vi "Extended.BuildSysexMsgI2CReadWrite.vi"(4 "use10BitsAddressMode?":bool, 6 "useAutoRestartTransmission?":bool, 7 "Read/Write Mode":T1(ring), 8 "error in":errorcluster, 9 "Register":u16 format="%.0x", 10 "I2C Write Data":u8[](array[numeric]) format="%x", 11 "Slave Address":u8 format="%x") -> (0 "error out":errorcluster, 1 "ReplyLength":i32=-1, 2 "ReplyFirstByte":T2=224 items=["ANALOG_IO_MESSAGE"=224, "DIGITAL_IO_MESSAGE"=144, "REPORT_ANALOG_PIN"=192, "REPORT_DIGITAL_PORT"=208, "START_SYSEX"=240, "END_SYSEX"=247, "SET_PIN_MODE"=244, "SET_DIGITAL_PIN_VALUE"=245, "PROTOCOL_VERSION"=249, "SYSTEM_RESET"=255, "SYSEX.EXTENDED_ID"=0, "SYSEX.RESERVED_USER_COMMANDs"=1, "SYSEX.ANALOG_MAPPING_QUERY"=105, "SYSEX.ANALOG_MAPPING_RESPONSE"=106, "SYSEX.CAPABILITY_QUERY"=107, "SYSEX.CAPABILITY_RESPONSE"=108, "SYSEX.PIN_STATE_QUERY"=109, "SYSEX.PIN_STATE_RESPONSE"=110, "SYSEX.REPORT_FIRMWARE"=121, "SYSEX.EXTENDED_ANALOG"=111, "SYSEX.STRING_DATA"=113, "SYSEX.REALTIME"=127, "SYSEX.NON_REALTIME"=126, "SYSEX.SAMPLING_INTERVAL"=122], 3 "I2CRequestMessage":u8[](array[numeric]) format="%x")   [LabVIEW 2020, in "FirmataClient.lvlib"]
doc: "Builds a message according to the Firmata Protocol Requirements. \n- https://github.com/firmata/protocol\n- https://github.com/firmata/protocol/blob/master/protocol.md"
uses:
  FirmataClient.lvlib
  controls/FirmataProtocolConstants.ctl
  8aab0f93-2f9c-4515-bdca-9512dbea522e.vi
  147f2e90-8315-44ff-bc99-ac74707c4f68.vi
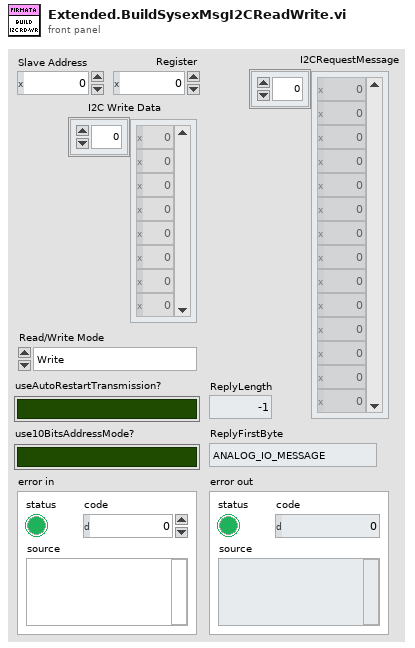
[diagram p1: front panel]
types:
  T1 = enum16{"Write", "Read Once", "Read Continuously", "Stop Continuous Reading"}
  T2 = typedef "FirmataClient.lvlib/FirmataProtocolConstants.ctl" = u16
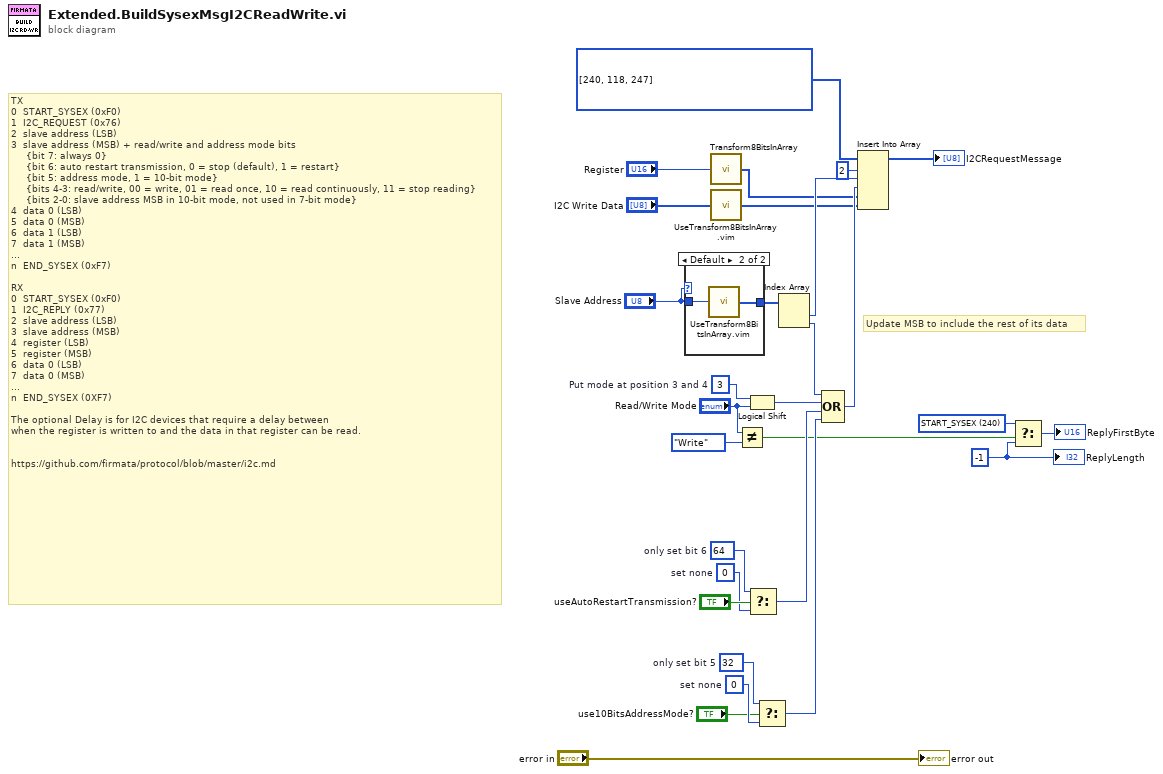
[diagram p0: block diagram]
diagram:
  w9 = T2 240 items=["ANALOG_IO_MESSAGE"=224, "DIGITAL_IO_MESSAGE"=144, "REPORT_ANALOG_PIN"=192, "REPORT_DIGITAL_PORT"=208, "START_SYSEX"=240, "END_SYSEX"=247, "SET_PIN_MODE"=244, "SET_DIGITAL_PIN_VALUE"=245, "PROTOCOL_VERSION"=249, "SYSTEM_RESET"=255, "SYSEX.EXTENDED_ID"=0, "SYSEX.RESERVED_USER_COMMANDs"=1, "SYSEX.ANALOG_MAPPING_QUERY"=105, "SYSEX.ANALOG_MAPPING_RESPONSE"=106, "SYSEX.CAPABILITY_QUERY"=107, "SYSEX.CAPABILITY_RESPONSE"=108, "SYSEX.PIN_STATE_QUERY"=109, "SYSEX.PIN_STATE_RESPONSE"=110, "SYSEX.REPORT_FIRMWARE"=121, "SYSEX.EXTENDED_ANALOG"=111, "SYSEX.STRING_DATA"=113, "SYSEX.REALTIME"=127, "SYSEX.NON_REALTIME"=126, "SYSEX.SAMPLING_INTERVAL"=122, "FEATURES.SYSEX.I2C_READ_WRITE"=118, "FEATURES.SYSEX.I2C_REPLY"=119, "FEATURES.SYSEX.I2C_CONFIG"=120] ("ReplyFirstByte")
  w16 = u8 0  # set none
  w15 = u8 32  # only set bit 5
  w18 = u8 0  # set none
  w19 = u8 64  # only set bit 6
  w11 = u8 3  # Put mode at position 3 and 4
  w8 = -1 ("ReplyLength")
  w27 = T2[] [240, 118, 247] items=["ANALOG_IO_MESSAGE"=224, "DIGITAL_IO_MESSAGE"=144, "REPORT_ANALOG_PIN"=192, "REPORT_DIGITAL_PORT"=208, "START_SYSEX"=240, "END_SYSEX"=247, "SET_PIN_MODE"=244, "SET_DIGITAL_PIN_VALUE"=245, "PROTOCOL_VERSION"=249, "SYSTEM_RESET"=255, "SYSEX.EXTENDED_ID"=0, "SYSEX.RESERVED_USER_COMMANDs"=1, "SYSEX.ANALOG_MAPPING_QUERY"=105, "SYSEX.ANALOG_MAPPING_RESPONSE"=106, "SYSEX.CAPABILITY_QUERY"=107, "SYSEX.CAPABILITY_RESPONSE"=108, "SYSEX.PIN_STATE_QUERY"=109, "SYSEX.PIN_STATE_RESPONSE"=110, "SYSEX.REPORT_FIRMWARE"=121, "SYSEX.EXTENDED_ANALOG"=111, "SYSEX.STRING_DATA"=113, "SYSEX.REALTIME"=127, "SYSEX.NON_REALTIME"=126, "SYSEX.SAMPLING_INTERVAL"=122, "FEATURES.SYSEX.I2C_READ_WRITE"=118, "FEATURES.SYSEX.I2C_REPLY"=119, "FEATURES.SYSEX.I2C_CONFIG"=120]
  # "Update MSB to include the rest of its data"
  # "TX\n0  START_SYSEX (0xF0)\n1  I2C_REQUEST (0x76)\n2  slave address (LSB)\n3  slave address (MSB) + read/write and address mode bits\n     {bit 7: always 0}\n     {bit 6: auto restart transmission, 0 = stop (default), 1 = restart}\n     {bit 5: address mode, 1 = 10-bit mode}\n     {bits 4-3: read/write, 00 = write, 01 = read once, 10 = read continuously, 11 = stop reading}\n     {bits 2-0: slave address MSB in 10-bit mode, not used in 7-bit mode}\n4  data 0 (LSB)\n5  data 0 (MSB)\n6  data 1 (LSB)\n7  data 1 (MSB)\n...\nn  END_SYSEX (0xF7)\n\nRX\n0  START_SYSEX (0xF0)\n1  I2C_REPLY (0x77)\n2  slave address (LSB)\n3  slave address (MSB)\n4  register (LSB)\n5  register (MSB)\n6  data 0 (LSB)\n7  data 0 (MSB)\n...\nn  END_SYSEX (0XF7)\n\nThe optional Delay is for I2C devices that require a delay between \nwhen the register is written to and the data in that register can be read.\n\n\nhttps://github.com/firmata/protocol/blob/master/i2c.md"
  n1 = case shown="Default" "Slave Address" {
    tunnel: "Slave Address" -> [_ w31]
    tunnel: [_ w30] -> w24
    frame ..0 {
    }
    frame Default {
      n2 = call "UseTransform8BitsInArray.vim"("Byte In"=w31) -> ("Byte Out"=w30:u32[])
    }
  }
  n3 = call "Transform8BitsInArray.vi"("Byte In"="Register") -> ("Byte Out"=w1:u32[])
  n4 = call "UseTransform8BitsInArray.vim"("Byte In"="I2C Write Data") -> ("Byte Out"=w2:u32[])
  n5 = Not Equal?(x="Read/Write Mode", y=T1."Write") -> (x != y?=w6:bool)
  n6 = Logical Shift(y=w11, x="Read/Write Mode") -> (x << y=w12:u32)
  n7 = Select(t=w19, s="useAutoRestartTransmission?", f=w18) -> (s? t:f=w17:u8)
  n8 = Select(t=w15, s="use10BitsAddressMode?", f=w16) -> (s? t:f=w13:u8)
  n9 = Index Array(array=w24) -> (element #1=w23:u32, element #2=w22:u32)  [unwired: 2 in]
  n10 = Compound Arithmetic op=OR(w22, w12, w17, w13) -> (w21:u32)
  n11 = Insert Into Array(array=w27, index=2, new element #1=w23, new element #2=w21, new element #3=w1, new element #4=w2) -> (→"I2CRequestMessage":T2[])
  n12 = Select(t=w9, s=w6, f=w8) -> (s? t:f=→"ReplyFirstByte":i32)
  "error out" <- "error in"
  "ReplyLength" <- w8
